vi "ControlCreate.vi"(0 "__args":T1) -> (2 "__errStatus":bool, 3 "__errCode":i32, 4 "__errSource":string)   [LabVIEW 2013]
uses:
  <vilib>/Utility/miscctls.llb/LVPointTypeDef.ctl
panel:
  out "__return":cluster{"UID":i32, "Terminal.UID":i32}
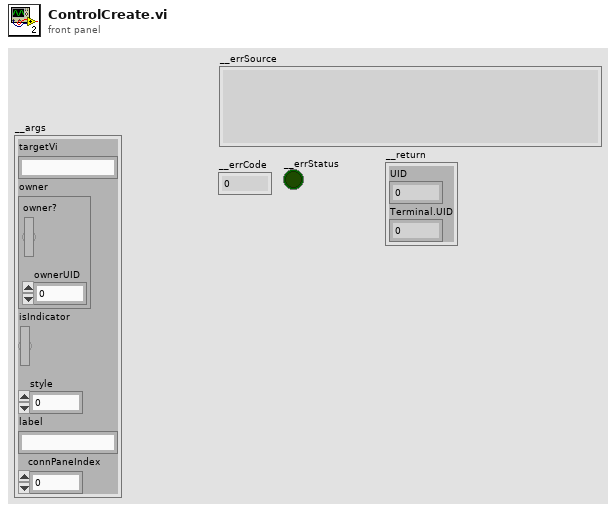
[diagram p1: front panel]
types:
  T1 = cluster{"targetVi":string, "owner":cluster{"owner?":bool, "ownerUID":i32}, "isIndicator":bool, "style":i32, "label":string, "connPaneIndex":i32}
  T2 = typedef "LVPointTypeDef.ctl" = cluster{"Horizontal":i16, "Vertical":i16}
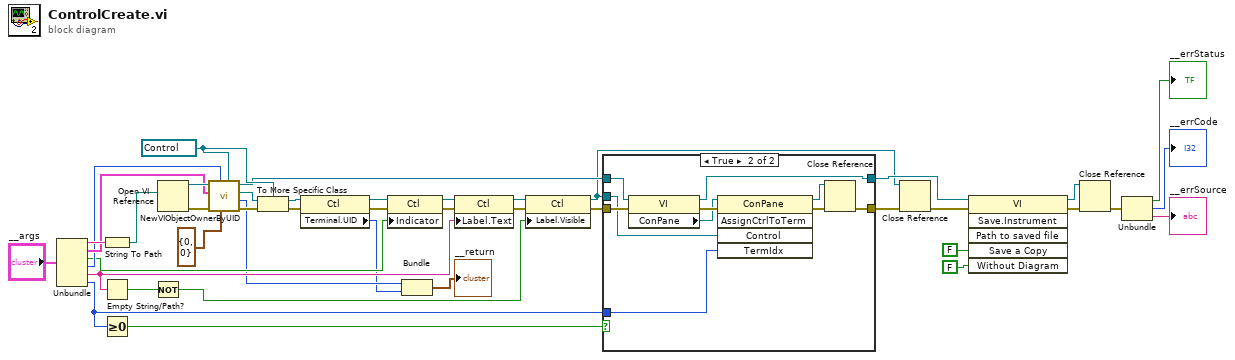
[diagram p0: block diagram]
diagram:
  w19 = refnum<vi> refnum ("vi object class")
  n1 = Unbundle("__args") -> ("targetVi"=w22:string, "owner"=w21:cluster{"owner?":bool, "ownerUID":i32}, "isIndicator"=w16:bool, "style"=w20:i32, "label"=w15:string, "connPaneIndex"=w1:i32)
  n2 = String To Path(string=w22) -> (path=w42:path)
  n3 = Empty String/Path?(string/path=w15) -> (empty?=w24:bool)
  n4 = Greater Or Equal To 0?(x=w1) -> (x >= 0?=w2:bool)
  n5 = Not(x=w24) -> (.not. x?=w25:bool)
  n6 = Open VI Reference(vi path=w42) -> (vi reference=w30:refnum<vi>, error out=w28:errorcluster)  [unwired: 5 in]
  n7 = call "NewVIObjectOwnerByUID.vi"("vi object class"=w19, "location"=T2 {"Horizontal"=0, "Vertical"=0}, "style"=w20, "error in (no error)"=w28, "owner"=w21, "targetVI"=w30) -> ("error out"=w27:errorcluster, "UID"=w10:i32, "object refnum"=w26:refnum<vi>, "dup targetVI"=w7:refnum<vi>)  [unwired: 2 in]
  n8 = To More Specific Class(target class=w19, reference=w26, error in=w27) -> (specific class reference=w12:refnum<vi>, error out=w14:errorcluster)
  n9 = property class="Ctl"(reference=w12, error in=w14) -> (reference out=w11:refnum<vi>, error out=w13:errorcluster, "Terminal.UID"=w9:i32)
  n10 = property class="Ctl"(reference=w11, error in=w13, "Indicator"=w16) -> (reference out=w18:refnum<vi>, error out=w17:errorcluster)
  n11 = Bundle("UID"=w10, "Terminal.UID"=w9) -> (→"__return":cluster{"UID":i32, "Terminal.UID":i32})  [unwired: 1 in]
  n12 = property class="Ctl"(reference=w18, error in=w17, "Label.Text"=w15) -> (reference out=w32:refnum<vi>, error out=w31:errorcluster)
  n13 = property class="Ctl"(reference=w32, error in=w31, "Label.Visible"=w25) -> (reference out=w3:refnum<vi>, error out=w6:errorcluster)
  n14 = case shown="True" w2 {
    tunnel: w7 -> [w44 w54]
    tunnel: w6 -> [w43 w53]
    tunnel: [w44 w52] -> w5
    tunnel: w1 -> [_ w49]
    tunnel: [w43 w47] -> w4
    tunnel: w3 -> [_ w45]
    frame False {
    }
    frame True {
      n15 = property class="VI"(reference=w54, error in=w53) -> (reference out=w52:refnum<vi>, error out=w51:errorcluster, "ConPane"=w50:refnum<vi>)
      n16 = invoke class="ConPane" method="AssignCtrlToTerm"(reference=w50, error in=w51, "Control"=w45, "TermIdx"=w49) -> (reference out=w48:refnum<vi>, error out=w46:errorcluster)  [unwired: 1 in, 3 out]
      n17 = Close Reference(reference=w48, error in (no error)=w46) -> (error out=w47:errorcluster)
    }
  }
  n18 = Close Reference(reference=w3, error in (no error)=w4) -> (error out=w36:errorcluster)
  n19 = invoke class="VI" method="Save.Instrument"(reference=w5, error in=w36, "Save a Copy"=FALSE, "Without Diagram"=FALSE) -> (reference out=w37:refnum<vi>, error out=w35:errorcluster)  [unwired: 2 in, 4 out]
  n20 = Close Reference(reference=w37, error in (no error)=w35) -> (error out=w38:errorcluster)
  n21 = Unbundle(w38) -> ("status"=→"__errStatus":bool, "code"=→"__errCode":i32, "source"=→"__errSource":string)
